vi "NI32LV210ASD6_parse_arduino_data_message (SubVI).vi"(9 "array type":dbl[](array[numeric]), 10 "data label":string, 11 "input string":string) -> (2 "array out":dbl[](array[numeric]), 3 "match length":i32)   [LabVIEW 2021]
uses:
  <vilib>/regexp/Match Regular Expression.xnode
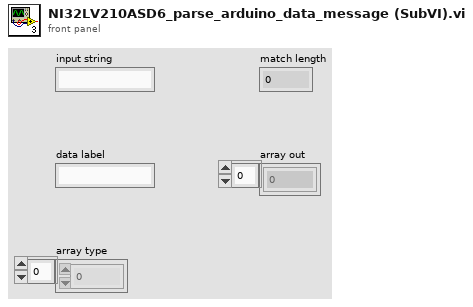
[diagram p1: front panel]
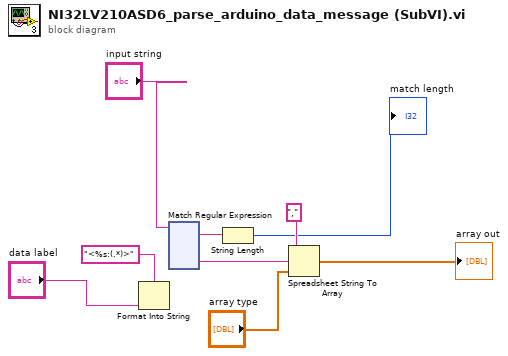
[diagram p0: block diagram]
diagram:
  n1 = Format Into String(format string="<%s:(.*)>", "data label") -> ()  [unwired: 2 in, 2 out]
  n2 = xnode "Match Regular Expression"("input string"="input string") -> ("whole match"=w2:string, "submatch 1"=w5:string)  [unwired: 5 in, 4 out]
  n3 = String Length(string=w2) -> (length=→"match length":i32)
  n4 = Spreadsheet String To Array(delimiter (Tab)=",", spreadsheet string=w5, array type (2D Dbl)="array type") -> (array=→"array out":dbl[])  [unwired: 1 in]
